vi "SGUpdateParameters.vi"(4 "SGAmp0":u16, 5 "SGSignalType0":u8, 6 "SGPhase0":u32, 7 "AOEnable0":bool, 8 "SGFreq0":u32, 9 "SGUpdateRate0":u32, 10 "AO0":i32, 11 "Refnum in":refnum<k21>) -> (3 "Refnum out":refnum<k21>)   [LabVIEW 2013, in "IRIO.lvlib"]
uses:
  IRIO.lvlib
  <vilib>/rvi/DataTransferAndStorage/Container/Common/niFpgaContainerExecOnDevCompGetState.vi
  <vilib>/rvi/DataTransferAndStorage/Register/Emulation/niFpgaRegisterEmulationFpgaImpl.vi
  <instcachedir>/0/niFpgaRegisterEmulationFpgaImpl_DCF4BC0110594B98B44A971D60CEEC4D.lvgen/niFpgaRegisterEmulationFpgaImpl_DCF4BC0110594B98B44A971D60CEEC4D_008.vi
  <vilib>/rvi/DataTransferAndStorage/Container/Common/niFpgaContainerGetUniqueNameForEmu.vi
  <vilib>/rvi/DataTransferAndStorage/Container/XNode/niFpgaContainer.xnode
  <vilib>/rvi/DataTransferAndStorage/Register/Emulation/niFpgaRegisterEmulationRefIn.vi
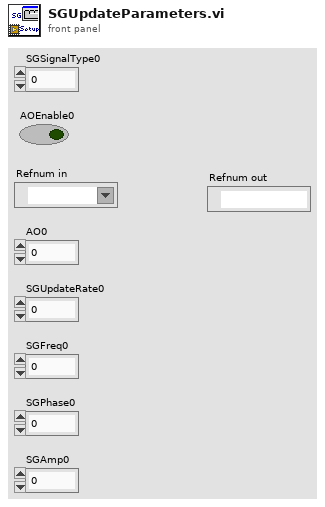
[diagram p1: front panel]
types:
  T1 = cluster{"AOEnable":bool, "AO0":i32, "SGUpdateRate":u32, "SGPhase":u32, "SGFreq":u32, "SGAmp":u16, "SGSignalType":u8, "N":u8}
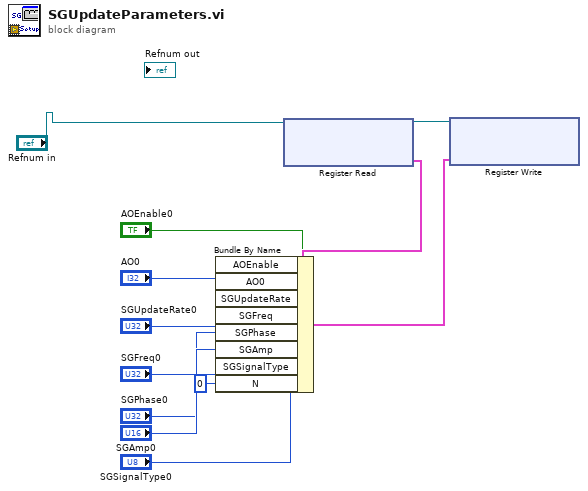
[diagram p0: block diagram]
diagram:
  n1 = xnode "Register Read"("Register In"="Refnum in") -> ("Data"=w12:T1, "Register Out"=w11:refnum<k21>)
  n2 = Bundle By Name(cluster=w12, "AOEnable"="AOEnable0", "AO0"="AO0", "SGUpdateRate"="SGUpdateRate0", "SGFreq"="SGFreq0", "SGPhase"="SGPhase0", "SGAmp"="SGAmp0", "SGSignalType"="SGSignalType0", "N"=u8 0) -> (w9:T1)
  n3 = xnode "Register Write"("Data"=w9, "Register In"=w11) -> ()  [unwired: 1 out]
